vi "SequenceEvent.PropertyChanged.vi"(4 "State":refnum<user-event>, 5 "Event Data":cluster{"sender":refnum<k24>, "e":refnum<k24>}, 6 "Control Ref":refnum<k24>, 7 "Event Common Data":T1) -> ()   [LabVIEW 2013, in "Simple Sequence Tools - Execution.lvlib"]
uses:
  NationalInstruments.VeriStand.RealTimeSequenceDefinitionApi
  Simple Sequence Tools - Execution.lvlib
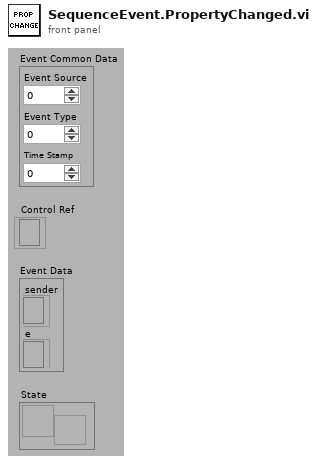
[diagram p1: front panel]
types:
  T1 = cluster{"Event Source":i32, "Event Type":u32, "Time Stamp":u32}
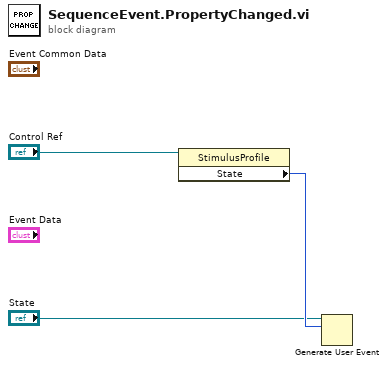
[diagram p0: block diagram]
diagram:
  n1 = property class="StimulusProfile"(reference="Control Ref") -> ("State"=w3:i32)  [unwired: 1 in, 2 out]
  n2 = Generate User Event(user event="State", event data cluster=w3) -> ()  [unwired: 2 in, 2 out]
